vi "ParserScaleType.vi"(8 "error in (no error)":errorcluster, 11 "JSON item":string) -> (0 "error out":errorcluster, 2 "Scale Type":T1, 3 "JSON item":string)   [LabVIEW 2017, in "Paser.lvlib"]
uses:
  Paser.lvlib
  <vilib>/JDP Science/JSONtext/JSONtext.lvlib
  Ctrl/ScaleType.ctl
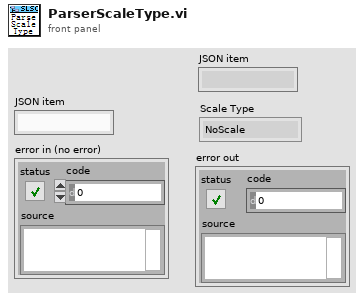
[diagram p1: front panel]
types:
  T1 = typedef "ScaleType.ctl" = enum16{"NoScale", "Table", "Polynomial", "Linear"}
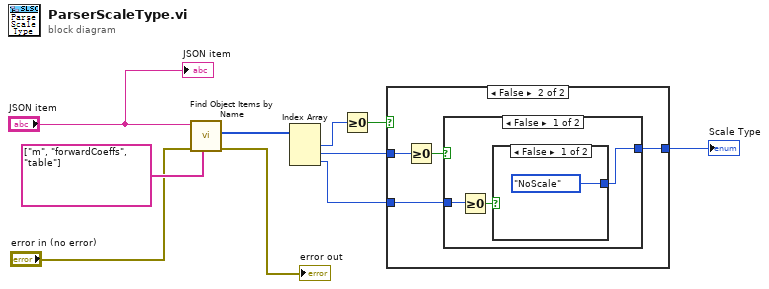
[diagram p0: block diagram]
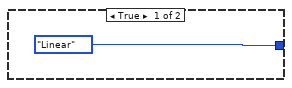
[diagram p2: hidden frame]
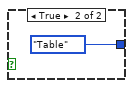
[diagram p3: hidden frame]
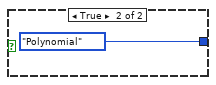
[diagram p4: hidden frame]
diagram:
  n1 = call <vilib>:"Find Object Items by Name.vi"("Item Names"=string[] ["m", "forwardCoeffs", "table"], "error in (no error)"="error in (no error)", "JSON"="JSON item") -> ("error out"=→"error out":errorcluster, "Offsets"=w6:i32[])  [unwired: 6 in, 1 out]
  n2 = Index Array(array=w6) -> (element #1=w7:i32, element #2=w9:i32, element #3=w10:i32)  [unwired: 3 in]
  n3 = Greater Or Equal To 0?(x=w7) -> (x >= 0?=w8:bool)
  n4 = case shown="False" w8 {
    tunnel: [ScaleType."Linear" w13] -> w1
    tunnel: w9 -> [_ w15]
    tunnel: w10 -> [_ w12]
    frame True {
    }
    frame False {
      n5 = Greater Or Equal To 0?(x=w15) -> (x >= 0?=w14:bool)
      n6 = case shown="False" w14 {
        tunnel: [w16 ScaleType."Polynomial"] -> w13
        tunnel: w12 -> [w18 _]
        frame False {
          n7 = Greater Or Equal To 0?(x=w18) -> (x >= 0?=w17:bool)
          n8 = case shown="False" w17 {
            tunnel: [ScaleType."NoScale" ScaleType."Table"] -> w16
            frame False {
            }
            frame True {
            }
          }
        }
        frame True {
        }
      }
    }
  }
  "Scale Type" <- w1
  "JSON item" <- "JSON item"
